vi "Delete Element at Index.vi"(0 "Variant (Cluster) in":variant, 7 "index":i32, 11 "error in (no error)":errorcluster) -> (4 "Variant (Cluster) out":variant, 6 "Name":string, 8 "element":variant, 15 "error out":errorcluster)   [LabVIEW 2017, in "Advanced Variant Tools.lvlib"]
uses:
  Advanced Variant Tools.lvlib
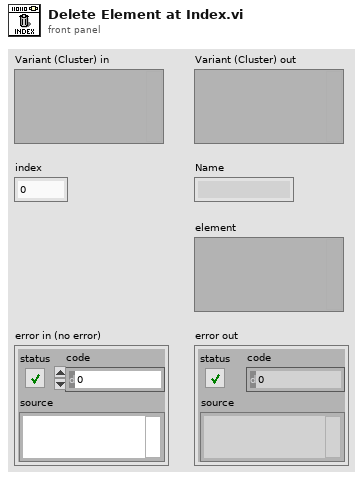
[diagram p1: front panel]
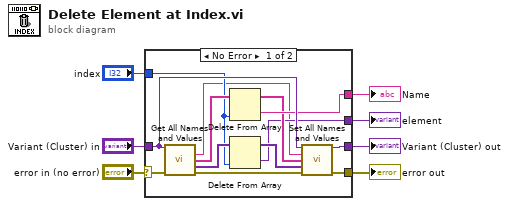
[diagram p0: block diagram]
diagram:
  n1 = case shown="No Error" "error in (no error)" {
    selector: "error in (no error)" -> [w20 w21]
    tunnel: [w17 w21] -> w6
    tunnel: [w16 w22] -> w5
    tunnel: "Variant (Cluster) in" -> [w15 w22]
    tunnel: [w13 _] -> w3
    tunnel: [w10 _] -> w2
    tunnel: "index" -> [w9 _]
    frame No Error {
      n2 = call "Get All Names and Values.vi"("Variant (Cluster) In"=w15, "error in"=w20) -> ("Name"=w8:string, "Element Names"=w14:string[], "Values"=w19:variant[], "error out"=w18:errorcluster)  [unwired: 9 in, 1 out]
      n3 = Delete From Array(array=w14, index=w9) -> (deleted portion=w13:string, array with subset deleted=w12:string[])  [unwired: 1 in]
      n4 = Delete From Array(array=w19, index=w9) -> (deleted portion=w10:variant, array with subset deleted=w11:variant[])  [unwired: 1 in]
      n5 = call "Set All Names and Values.vi"("Variant (Cluster) In"=w15, "Name"=w8, "Element Names"=w12, "values"=w11, "error in"=w18) -> ("Variant (Cluster) Out"=w16:variant, "error out"=w17:errorcluster)  [unwired: 9 in]
    }
    frame Error {
    }
  }
  "Variant (Cluster) out" <- w5
  "error out" <- w6
  "element" <- w2
  "Name" <- w3
